vi "Main.vi"(10 "VISA resource name":refnum<visa-resource-name>, 11 "Module Admin":refnum<class "Delacor_lib_QMH_Cloneable Module Admin.lvclass">) -> ()   [LabVIEW 2018, in "Clonable_test.lvlib"]
doc: "This template is based off of the Queued Message Handler design pattern and the Queued Message Handler project template that ships with LabVIEW.\n\nThe main difference is that the queue is private to this module and communication between modules is performed via Broadcast and Request events.\n\nRequest events are wrapped in public API methods and are handled in the Event Handling Loop (EHL) of this VI. Any module can register for Broadcast events sent by this module. The EHL generates messages based on user interface actions.\n\nThe Message Handling Loop (MHL) processes messages generated by the EHL, or by other messages. The messages are string values, so new messages can be added easily to the Message Cases case structure in the MHL. Each message cluster can also provide an optional value for Message Data, which is a variant that can be converted to whatever message-specific data is required.\n_____\nBased on DQMH Project Template 6.0.0.91."
uses:
  Clonable_test.lvlib
  <vilib>/Delacor/Delacor QMH/Libraries/Cloneable Module Admin_class/Delacor_lib_QMH_Cloneable Module Admin.lvclass
  C:/Program Files (x86)/National Instruments/LabVIEW 2018/vi.lib/Delacor/Delacor QMH/Libraries/Module Admin_class/Delacor_lib_QMH_Module Admin.lvclass
  Module Data--cluster.ctl
  <vilib>/Delacor/Delacor QMH/Libraries/Message Queue_class/Delacor_lib_QMH_Message Queue.lvclass/Delacor_lib_QMH_Message Queue.ctl
  <vilib>/Delacor/Delacor QMH/Libraries/Cloneable Module Admin_class/Delacor_lib_QMH_Cloneable Module Admin.lvclass/Delacor_lib_QMH_Cloneable Module Admin.ctl
  Stop Argument--cluster.ctl
  <vilib>/Delacor/Delacor QMH/Libraries/Module Admin_class/Delacor_lib_QMH_Module Admin.lvclass/Delacor_lib_QMH_Module Admin.ctl
  Get data from module Argument--cluster.ctl
  Get data from module (Reply Payload)--cluster.ctl
  start send Argument--cluster.ctl
  stop send Argument--cluster.ctl
  <vilib>/Utility/miscctls.llb/LVPointTypeDef.ctl
  <vilib>/Delacor/Delacor QMH/Libraries/Message Queue_class/Delacor_lib_QMH_Enqueue Message (Single).vi
  <vilib>/Delacor/Delacor QMH/Libraries/Cloneable Module Admin_class/Delacor_lib_QMH_Get Module ID.vi
  <vilib>/Delacor/Delacor QMH/Libraries/Module Admin_class/Delacor_lib_QMH_Get External Launch.vi
  <vilib>/Utility/error.llb/Error Cluster From Error Code.vi
  <vilib>/ErrorRing/Error Ring.xnode
  <vilib>/Delacor/Delacor QMH/Libraries/Message Queue_class/Delacor_lib_QMH_Message Queue.lvclass
panel:
  out "error out":errorcluster
  out "Status":string
  in  "Simulate EHL Error":bool
  in  "Simulate MHL Error":bool
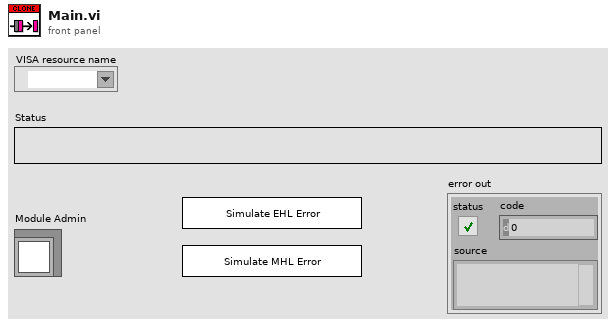
[diagram p1: front panel]
types:
  T1 = typedef "Clonable_test.lvlib/Request Events--cluster.ctl" = cluster{"Stop Module":refnum<user-event>, "Show Panel":refnum<user-event>, "Hide Panel":refnum<user-event>, "Show Diagram":refnum<user-event>, "Get Module Execution Status":refnum<user-event>, "Get data from module":refnum<user-event>, "start send":refnum<user-event>, "stop send":refnum<user-event>}
  T2 = typedef "Clonable_test.lvlib/Module Data--cluster.ctl" = cluster{"Status":string, "VISA resource name":refnum<visa-resource-name>}
  T3 = enum32{"invalid lock state", "Not Locked", "Locked (No Password)", "Password-protected"}
  T4 = typedef "Clonable_test.lvlib/Stop Argument--cluster.ctl" = cluster{"Module ID":i32, "Origin":string, "Exit via Stop Module Req?":bool, "Wait for Module to stop?":bool}
  T5 = typedef "Clonable_test.lvlib/Get data from module Argument--cluster.ctl" = cluster{"Module ID":i32, "Wait Notifier":refnum<notifier>, "wait for reply":bool}
  T6 = typedef "Clonable_test.lvlib/start send Argument--cluster.ctl" = cluster{"Module ID":i32, "Boolean":bool}
  T7 = typedef "Clonable_test.lvlib/stop send Argument--cluster.ctl" = cluster{"Module ID":i32, "Boolean":bool}
  T8 = typedef "LVPointTypeDef.ctl" = cluster{"Horizontal":i16, "Vertical":i16}
  T9 = enum32{"Invalid", "Standard", "Closed", "Hidden", "Minimized", "Maximized"}
  T10 = typedef "Clonable_test.lvlib/Get data from module (Reply Payload)--cluster.ctl" = cluster{"String":string, "Get data from module_error":errorcluster}
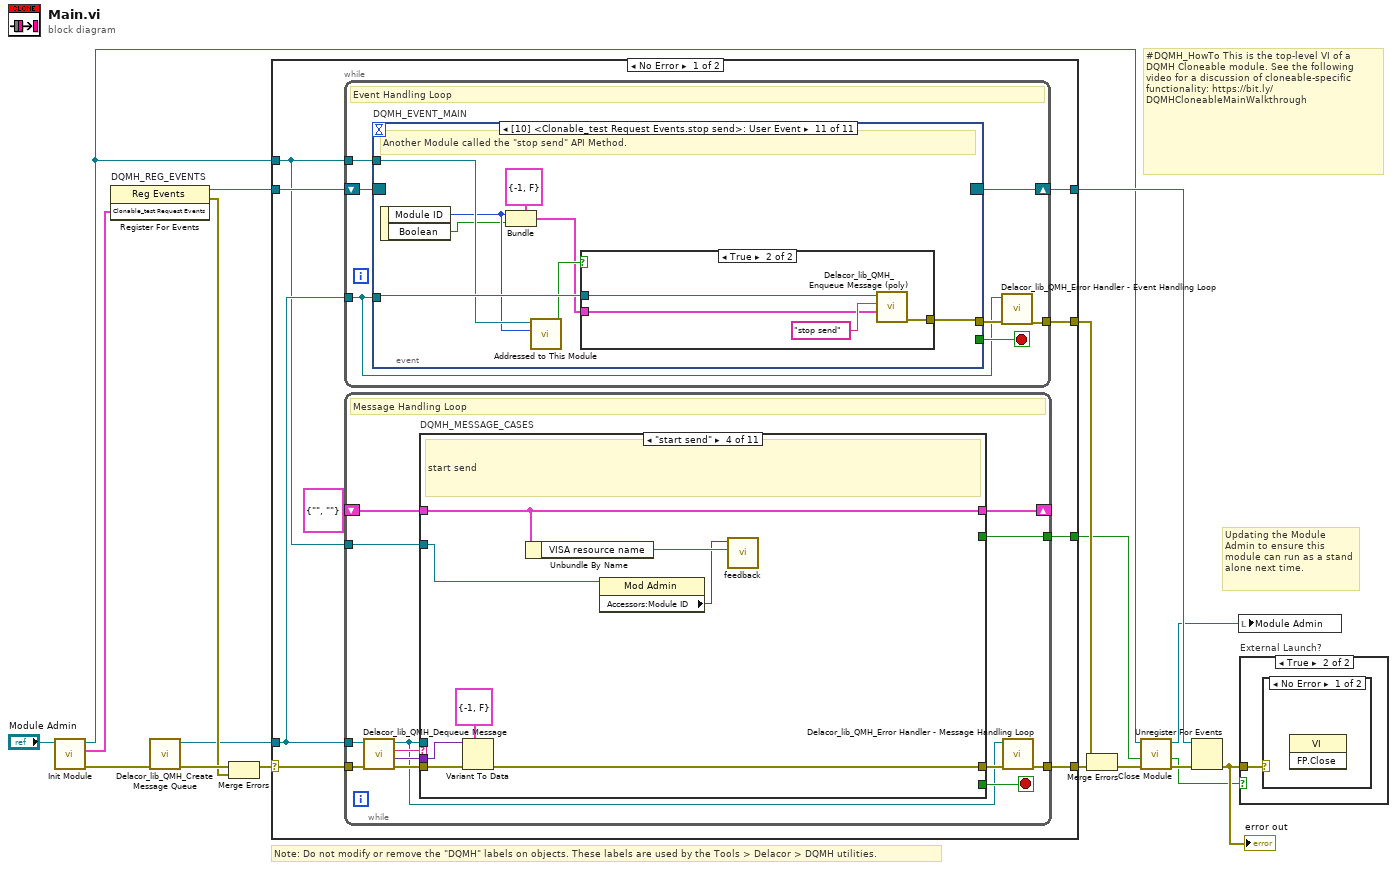
[diagram p0: block diagram]
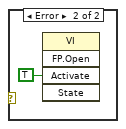
[diagram p3: hidden frame]
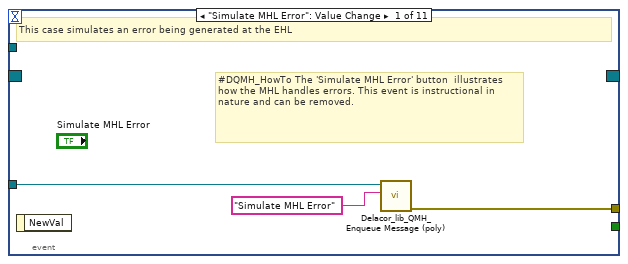
[diagram p4: hidden frame]
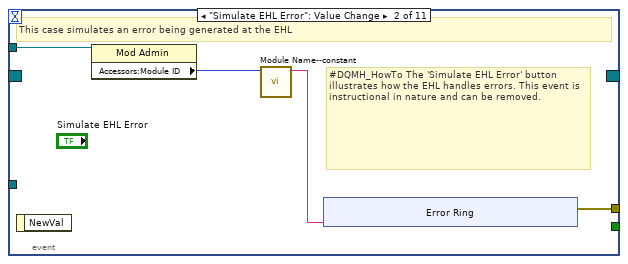
[diagram p5: hidden frame]
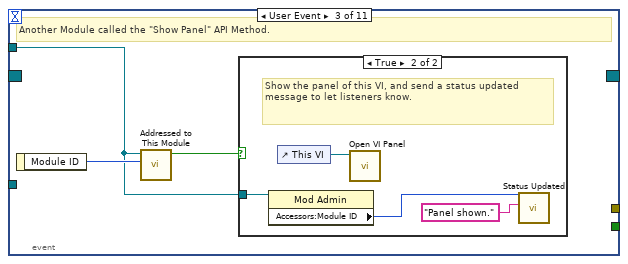
[diagram p6: hidden frame]
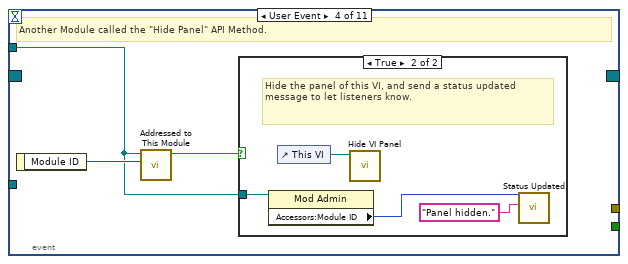
[diagram p8: hidden frame]
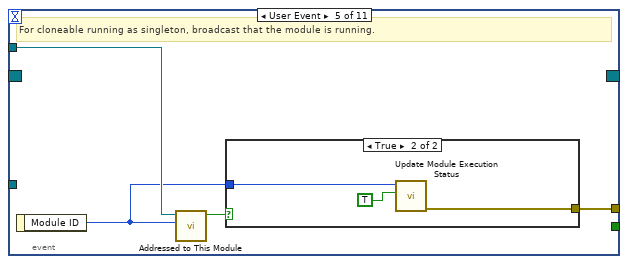
[diagram p10: hidden frame]
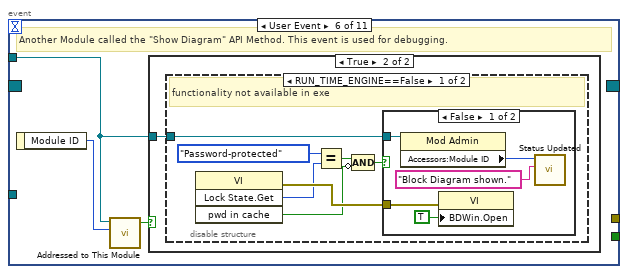
[diagram p12: hidden frame]
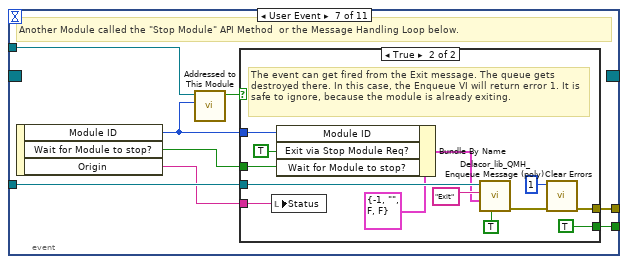
[diagram p16: hidden frame]
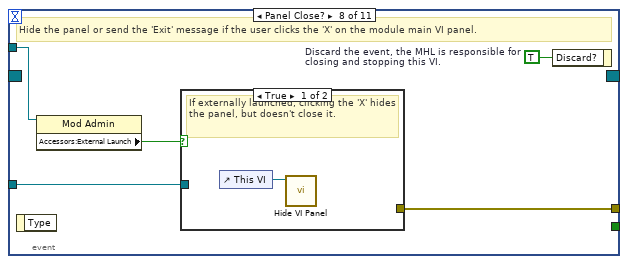
[diagram p18: hidden frame]
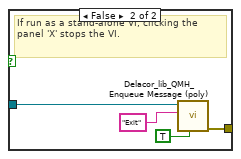
[diagram p19: hidden frame]
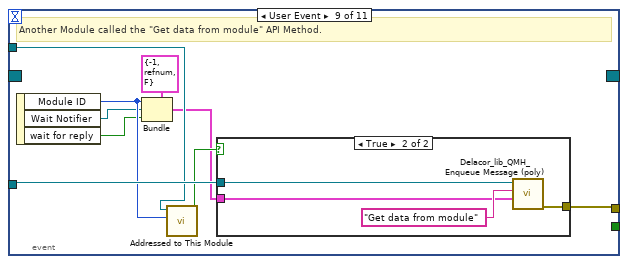
[diagram p20: hidden frame]
diagram:
  # "#DQMH_HowTo This is the top-level VI of a DQMH Cloneable module. See the following video for a discussion of cloneable-specific functionality: https://bit.ly/DQMHCloneableMainWalkthrough"
  # "Note: Do not modify or remove the \"DQMH\" labels on objects. These labels are used by the Tools > Delacor > DQMH utilities."
  # "Updating the Module Admin to ensure this module can run as a stand alone next time."
  n1 = call "Init Module.vi"("Cloneable Module Admin in"="Module Admin") -> ("error out"=w15:errorcluster, "Clonable_test Request Events"=w7:T1, "Cloneable Module Admin out"=w4:refnum<class "Delacor_lib_QMH_Cloneable Module Admin.lvclass">)  [unwired: 8 in]
  n2 = register-events "DQMH_REG_EVENTS"(w7) -> (reference out=w8:refnum<event-registration>, error out=w10:errorcluster)  [unwired: 2 in]
  n3 = call <vilib>:"Delacor_lib_QMH_Create Message Queue.vi"("error in"=w15) -> ("error out"=w12:errorcluster, "Message Queue"=w6:refnum<class "Delacor_lib_QMH_Message Queue.lvclass">)  [unwired: 9 in]
  n4 = Merge Errors(w12, w10) -> (w11:errorcluster)
  n5 = case shown="No Error" w11 {
    selector: w11 -> [w25 w296]
    tunnel: [w27 w295] -> w16
    tunnel: [w24 w303] -> w9
    tunnel: w8 -> [w22 w303]
    tunnel: w6 -> [w21 w294]
    tunnel: [w26 _] -> w17
    tunnel: w4 -> [w20 w299]
    tunnel: [w19 _] -> w2
    frame No Error {
      n6 = while {
        tunnel: w21 -> [w28]
        shift-right: [w31] -> w24
        shift-left: w22 -> [w32]
        tunnel: [w33] -> w26
        tunnel: w20 -> [w29]
        stop <- w30 stop-if-true
        # "Event Handling Loop"
        n7 = event "DQMH_EVENT_MAIN" shown="[10] <Clonable_test Request Events.stop send>: User Event" {
          selector: w32 -> [_ _ _ _ _ _ _ _ _ _ _]
          dyn-events: [_ _ _ _ _ _ _ _ _ _ _] -> w31
          timeout: _ -> [_ _ _ _ _ _ _ _ _ _ _]
          tunnel: [_ _ _ _ _ _ w89 _ _ _ _] -> w30
          tunnel: w28 -> [w36 _ _ _ _ _ w92 w108 w125 w137 w149]
          tunnel: [w37 w41 _ _ w66 _ w93 w111 w117 w130 w142] -> w34
          tunnel: w29 -> [_ w40 w49 w56 w64 w70 w91 w109 w123 w135 w147]
          event "Simulate MHL Error": Value Change {
            # "#DQMH_HowTo The 'Simulate MHL Error' button  illustrates how the MHL handles errors. This event is instructional in nature and can be removed."
            # "This case simulates an error being generated at the EHL"
            n8 = event-data() -> ()  [unwired: 1 in, 1 out]
            n9 = call-poly <vilib>:"Delacor_lib_QMH_Enqueue Message (poly).vi"("Message"="Simulate MHL Error", "Message Queue in"=w36) -> ("error out"=w37:errorcluster)  [unwired: 8 in, 1 out]
          }
          event "Simulate EHL Error": Value Change {
            # "#DQMH_HowTo The 'Simulate EHL Error' button  illustrates how the EHL handles errors. This event is instructional in nature and can be removed."
            # "This case simulates an error being generated at the EHL"
            n10 = event-data() -> ()  [unwired: 1 in, 1 out]
            n11 = property class="Mod Admin"(reference=w40) -> ("Accessors:Module ID"=w39:i32)  [unwired: 1 in, 2 out]
            n12 = call "Module Name--constant.vi"("Module ID"=w39) -> ("Module Name"=w38:string)  [unwired: 10 in]
            n13 = xnode "Error Ring"("parameter 0"=w38) -> ("error out"=w41:errorcluster)
          }
          event User Event {
            # "Another Module called the \"Show Panel\" API Method."
            n14 = event-data() -> ("Module ID"=w50:i32)  [unwired: 1 in]
            n15 = call "Addressed to This Module.vi"("Module ID from Argument"=w50, "Module Admin"=w49) -> ("Addressed to this instance?"=w51:bool)  [unwired: 8 in, 1 out]
            n16 = case shown="True" w51 {
              tunnel: w49 -> [_ w53]
              frame False {
              }
              frame True {
                # "Show the panel of this VI, and send a status updated message to let listeners know."
                n17 = property class="Mod Admin"(reference=w53) -> ("Accessors:Module ID"=w52:i32)  [unwired: 1 in, 2 out]
                n18 = control-ref of="This VI"() -> (w55:refnum<vi>)
                n19 = call "Open VI Panel.vi"("VI"=w55) -> ()  [unwired: 10 in, 1 out]
                n20 = call "Status Updated.vi"("Status"="Panel shown." ("format string"), "Module ID"=w52) -> ()  [unwired: 9 in, 1 out]
              }
            }
          }
          event User Event {
            # "Another Module called the \"Hide Panel\" API Method."
            n21 = event-data() -> ("Module ID"=w57:i32)  [unwired: 1 in]
            n22 = call "Addressed to This Module.vi"("Module ID from Argument"=w57, "Module Admin"=w56) -> ("Addressed to this instance?"=w58:bool)  [unwired: 8 in, 1 out]
            n23 = case shown="True" w58 {
              tunnel: w56 -> [_ w60]
              frame False {
              }
              frame True {
                # "Hide the panel of this VI, and send a status updated message to let listeners know."
                n24 = property class="Mod Admin"(reference=w60) -> ("Accessors:Module ID"=w59:i32)  [unwired: 1 in, 2 out]
                n25 = control-ref of="This VI"() -> (w62:refnum<vi>)
                n26 = call "Hide VI Panel.vi"("VI"=w62) -> ()  [unwired: 10 in, 1 out]
                n27 = call "Status Updated.vi"("Status"="Panel hidden." ("format string"), "Module ID"=w59) -> ()  [unwired: 9 in, 1 out]
              }
            }
          }
          event User Event {
            # "For cloneable running as singleton, broadcast that the module is running."
            n28 = event-data() -> ("Module ID"=w63:i32)  [unwired: 1 in]
            n29 = call "Addressed to This Module.vi"("Module ID from Argument"=w63, "Module Admin"=w64) -> ("Addressed to this instance?"=w65:bool)  [unwired: 8 in, 1 out]
            n30 = case shown="True" w65 {
              tunnel: [_ w69] -> w66
              tunnel: w63 -> [_ w68]
              frame False {
              }
              frame True {
                n31 = call "Update Module Execution Status.vi"("Running?"=TRUE, "Module ID"=w68) -> ("error out"=w69:errorcluster)  [unwired: 9 in]
              }
            }
          }
          event User Event {
            # "Another Module called the \"Show Diagram\" API Method. This event is used for debugging."
            n32 = event-data() -> ("Module ID"=w71:i32)  [unwired: 1 in]
            n33 = call "Addressed to This Module.vi"("Module ID from Argument"=w71, "Module Admin"=w70) -> ("Addressed to this instance?"=w72:bool)  [unwired: 8 in, 1 out]
            n34 = case shown="True" w72 {
              tunnel: w70 -> [_ w73]
              frame False {
              }
              frame True {
                n35 = disable-structure shown="RUN_TIME_ENGINE==False" {
                  disable-tunnel: w73 -> [w74 _]
                  frame condition #0 (active) {
                    # "functionality not available in exe"
                    n36 = invoke class="VI" method="Lock State.Get"() -> (error out=w80:errorcluster, "Get Lock State"=w79:T3, "pwd in cache"=w76:bool)  [unwired: 4 in, 1 out]
                    n37 = Equal?(x=T3."Password-protected", y=w79) -> (x = y?=w77:bool)
                    n38 = Compound Arithmetic op=AND(w77, invert w76) -> (w75:bool)
                    n39 = case shown="False" w75 {
                      tunnel: w80 -> [w85 _]
                      tunnel: w74 -> [w82 _]
                      frame False {
                        n40 = property class="Mod Admin"(reference=w82) -> ("Accessors:Module ID"=w81:i32)  [unwired: 1 in, 2 out]
                        n41 = property class="VI"(error in=w85, "BDWin.Open"=TRUE ("Block Diagram Window:Open")) -> ()  [unwired: 1 in, 2 out]
                        n42 = call "Status Updated.vi"("Status"="Block Diagram shown." ("format string"), "Module ID"=w81) -> ()  [unwired: 9 in, 1 out]
                      }
                      frame True {
                        # "Password-protected VI, and the password is not in the cache. Do not show the diagram."
                      }
                    }
                  }
                  frame condition #1 {
                  }
                }
              }
            }
          }
          event User Event {
            # "Another Module called the \"Stop Module\" API Method  or the Message Handling Loop below."
            n43 = event-data() -> ("Module ID"=w87:i32, "Wait for Module to stop?"=w88:bool, "Origin"=w86:string)  [unwired: 1 in]
            n44 = call "Addressed to This Module.vi"("Module ID from Argument"=w87, "Module Admin"=w91) -> ("Addressed to this instance?"=w90:bool)  [unwired: 8 in, 1 out]
            n45 = case shown="True" w90 {
              tunnel: [_ w105] -> w93
              tunnel: w92 -> [_ w101]
              tunnel: [_ TRUE] -> w89
              tunnel: w88 -> [_ w96]
              tunnel: w87 -> [_ w98]
              tunnel: w86 -> [_ w94]
              frame False {
              }
              frame True {
                # "The event can get fired from the Exit message. The queue gets destroyed there. In this case, the Enqueue VI will return error 1. It is safe to ignore, because the module is already exiting."
                n46 = local write "Status"(w94) -> ()
                n47 = Bundle By Name(cluster=T4 {"Module ID"=-1, "Origin"="", "Exit via Stop Module Req?"=FALSE, "Wait for Module to stop?"=FALSE} ("Stop Argument"), "Module ID"=w98, "Exit via Stop Module Req?"=TRUE, "Wait for Module to stop?"=w96) -> (w95:T4)
                n48 = call-poly <vilib>:"Delacor_lib_QMH_Enqueue Message (poly).vi"("Priority Message? (F)"=TRUE, "Message Data"=w95, "Message"="Exit", "Message Queue in"=w101) -> ("error out"=w106:errorcluster)  [unwired: 6 in, 1 out]
                n49 = call <vilib>:"Clear Errors.vi"("error in (no error)"=w106, "specific error code to clear (0: all)"=1) -> ("error out"=w105:errorcluster)  [unwired: 4 in, 1 out]
              }
            }
          }
          event Panel Close? {
            w110 = TRUE  # Discard the event, the MHL is responsible for closing and stopping this VI.
            # "Hide the panel or send the 'Exit' message if the user clicks the 'X' on the module main VI panel."
            n50 = event-data() -> ()  [unwired: 1 in, 1 out]
            n51 = property class="Mod Admin"(reference=w109) -> ("Accessors:External Launch"=w107:bool)  [unwired: 1 in, 2 out]
            n52 = case shown="True" w107 {
              tunnel: w108 -> [_ w115]
              tunnel: [_ w116] -> w111
              frame True {
                # "If externally launched, clicking the 'X' hides the panel, but doesn't close it."
                n53 = control-ref of="This VI"() -> (w112:refnum<vi>)
                n54 = call "Hide VI Panel.vi"("VI"=w112) -> ()  [unwired: 10 in, 1 out]
              }
              frame False {
                # "If run as a stand-alone VI, clicking the panel 'X' stops the VI."
                n55 = call-poly <vilib>:"Delacor_lib_QMH_Enqueue Message (poly).vi"("Priority Message? (F)"=TRUE, "Message"="Exit", "Message Queue in"=w115) -> ("error out"=w116:errorcluster)  [unwired: 7 in, 1 out]
              }
            }
            n56 = event-data("Discard?"=w110) -> ()  [unwired: 1 in, 1 out]
          }
          event User Event {
            # "Another Module called the \"Get data from module\" API Method."
            n57 = event-data() -> ("Module ID"=w120:i32, "Wait Notifier"=w119:refnum<notifier>, "wait for reply"=w118:bool)  [unwired: 1 in]
            n58 = Bundle(cluster=T5 {"Module ID"=-1, "Wait Notifier"=refnum, "wait for reply"=FALSE} ("Get data from module Argument"), "Module ID"=w120, "Wait Notifier"=w119, "wait for reply"=w118) -> (w121:T5)
            n59 = call "Addressed to This Module.vi"("Module ID from Argument"=w120, "Module Admin"=w123) -> ("Addressed to this instance?"=w124:bool)  [unwired: 8 in, 1 out]
            n60 = case shown="True" w124 {
              tunnel: w125 -> [_ w129]
              tunnel: w121 -> [_ w127]
              tunnel: [_ w126] -> w117
              frame False {
              }
              frame True {
                n61 = call-poly <vilib>:"Delacor_lib_QMH_Enqueue Message (poly).vi"("Message Data"=w127, "Message"="Get data from module", "Message Queue in"=w129) -> ("error out"=w126:errorcluster)  [unwired: 7 in, 1 out]
              }
            }
          }
          event User Event {
            # "Another Module called the \"start send\" API Method."
            n62 = event-data() -> ("Module ID"=w132:i32, "Boolean"=w131:bool)  [unwired: 1 in]
            n63 = Bundle(cluster=T6 {"Module ID"=-1, "Boolean"=FALSE} ("start send Argument"), "Module ID"=w132, "Boolean"=w131) -> (w133:T6)
            n64 = call "Addressed to This Module.vi"("Module ID from Argument"=w132, "Module Admin"=w135) -> ("Addressed to this instance?"=w136:bool)  [unwired: 8 in, 1 out]
            n65 = case shown="True" w136 {
              tunnel: w137 -> [_ w141]
              tunnel: w133 -> [_ w139]
              tunnel: [_ w138] -> w130
              frame False {
              }
              frame True {
                n66 = call-poly <vilib>:"Delacor_lib_QMH_Enqueue Message (poly).vi"("Message Data"=w139, "Message"="start send", "Message Queue in"=w141) -> ("error out"=w138:errorcluster)  [unwired: 7 in, 1 out]
              }
            }
          }
          event User Event {
            # "Another Module called the \"stop send\" API Method."
            n67 = event-data() -> ("Module ID"=w144:i32, "Boolean"=w143:bool)  [unwired: 1 in]
            n68 = Bundle(cluster=T7 {"Module ID"=-1, "Boolean"=FALSE} ("stop send Argument"), "Module ID"=w144, "Boolean"=w143) -> (w145:T7)
            n69 = call "Addressed to This Module.vi"("Module ID from Argument"=w144, "Module Admin"=w147) -> ("Addressed to this instance?"=w148:bool)  [unwired: 8 in, 1 out]
            n70 = case shown="True" w148 {
              tunnel: w149 -> [_ w153]
              tunnel: w145 -> [_ w151]
              tunnel: [_ w150] -> w142
              frame False {
              }
              frame True {
                n71 = call-poly <vilib>:"Delacor_lib_QMH_Enqueue Message (poly).vi"("Message Data"=w151, "Message"="stop send", "Message Queue in"=w153) -> ("error out"=w150:errorcluster)  [unwired: 7 in, 1 out]
              }
            }
          }
        }
        n72 = call-dynamic "Delacor_lib_QMH_Error Handler - Event Handling Loop.vi"("error in"=w34, "Message Queue in"=w28) -> ("dup error in"=w33:errorcluster)  [unwired: 8 in, 1 out]
      }
      n73 = while {
        tunnel: w21 -> [w157]
        shift-right: [w161] -> _
        shift-left: T2 {"Status"="", "VISA resource name"=""} ("Data Cluster") -> [w162]
        tunnel: w25 -> [w165]
        tunnel: [w163] -> w27
        tunnel: w20 -> [w155]
        tunnel: [w154] -> w19
        stop <- w160 stop-if-true
        # "Message Handling Loop"
        n74 = call-dynamic "Delacor_lib_QMH_Dequeue Message.vi"("error in"=w165, "Message Queue in"=w157) -> ("error out"=w164:errorcluster, "Message Data"=w158:variant, "Message"=w159:string, "Message Queue out"=w156:refnum<class "Delacor_lib_QMH_Message Queue.lvclass">)  [unwired: 6 in]
        n75 = case "DQMH_MESSAGE_CASES" shown="\"start send\"" w159 {
          selector: w159 -> [_ _ _ _ _ _ _ _ _ _ w281]
          tunnel: w156 -> [_ _ _ _ _ _ _ w232 _ w271 _]
          tunnel: w164 -> [w187 w191 w209 w219 w225 w228 w230 w241 w254 w277 w283]
          tunnel: [w185 w191 w200 w218 w223 w227 w230 w237 w253 w274 w284] -> w166
          tunnel: w162 -> [w167 w190 w197 w215 w224 w226 w229 w236 w251 w270 w282]
          tunnel: [w178 w190 w197 w215 w224 w226 w229 w236 w251 w270 w282] -> w161
          tunnel: [_ _ _ _ _ _ _ _ _ w269 _] -> w160
          tunnel: w158 -> [_ _ w207 w217 w222 _ _ w235 _ w267 _]
          tunnel: w155 -> [w173 _ _ w213 _ _ _ w234 w249 w263 w279]
          tunnel: [_ _ _ _ _ _ _ _ _ w265 _] -> w154
          frame "Initialize" {
            w170 = "Initial Message" ("Initial Message")
            # "Initialize - Any operation that needs to be done before the module can receive messages. Synchronize Caller Events.vi will inform Start Module.vi that the module has launched and is ready to receive messages. Module Did Init.vi will broadcast that the module initialized."
            n76 = call "Synchronize Caller Events.vi"("error in (no error)"=w187, "Module Admin"=w173) -> ("error out"=w186:errorcluster, "Module Admin out"=w172:refnum<class "Delacor_lib_QMH_Cloneable Module Admin.lvclass">)  [unwired: 8 in]
            n77 = property class="Mod Admin"(reference=w172) -> ("Accessors:Module ID"=w175:i32, "Accessors:External Launch"=w174:bool)  [unwired: 1 in, 2 out]
            n78 = Bundle By Name(cluster=w167, "VISA resource name"="VISA resource name") -> (w168:T2)
            n79 = call "Module Name--constant.vi"("Module ID"=w175) -> ("Module Name"=w182:string)  [unwired: 10 in]
            n80 = property class="VI"("Front Panel.Title"=w182) -> (reference out=w184:refnum<vi>, error out=w189:errorcluster)  [unwired: 2 in]
            n81 = Select(t=T9."Hidden" ("State"), s=w174, f=T9."Standard" ("State")) -> (s? t:f=w179:T9)
            n82 = invoke class="VI" method="FP.Open"(reference=w184, error in=w189, "State"=w179) -> (reference out=w183:refnum<vi>, error out=w188:errorcluster)  [unwired: 2 in, 3 out]
            n83 = call "Module Name--constant.vi"("Module ID"=w175) -> ("Module Name"=w176:string)  [unwired: 10 in]
            n84 = Bundle By Name(cluster=w168, "Status"=w170) -> (w178:T2)
            n85 = invoke class="VI" method="FP.Center"(reference=w183, error in=w188) -> ()  [unwired: 1 in, 3 out]
            n86 = property on="Pane" class="Pane"("Origin"=T8 {"Horizontal"=0, "Vertical"=0}) -> ()  [unwired: 2 in, 2 out]
            n87 = call "Module Did Init.vi"("error in (no error)"=w186, "Initialized?"=TRUE, "Origin"=w176, "Module ID"=w175) -> ("error out"=w185:errorcluster)  [unwired: 7 in]
            "Status" <- w170
          }
          frame "---Module Specific---" {
            # "Separator -- The following cases handle messages specific to this Module."
          }
          frame "Get data from module" {
            # "test function get data from each module"
            n88 = Unbundle By Name(w197) -> ("VISA resource name"=w195:refnum<visa-resource-name>)
            n89 = Variant To Data(error in=w209, type=T5 {"Module ID"=-1, "Wait Notifier"=refnum, "wait for reply"=FALSE} ("Get data from module Argument"), Variant=w207) -> (data=w205:T5, error out=w208:errorcluster)
            n90 = feedback #1(0) -> (w199:i32)
            n91 = Increment(x=w199) -> (x+1=w194:i32)
            n92 = feedback-in #1(w194) -> ()
            n93 = Unbundle By Name(w205) -> ("Wait Notifier"=w204:refnum<notifier>, "wait for reply"=w203:bool)  [unwired: 1 out]
            n94 = Format Into String(format string="%d: %s\\n", w194, w195) -> (resulting string=w193:string, error out=w192:errorcluster)  [unwired: 2 in]
            n95 = Bundle By Name(cluster=T10 {"String"="", "Get data from module_error"={"status"=FALSE, "code"=0, "source"=""}} ("Get data from module (Reply Payload)"), "String"=w193, "Get data from module_error"=w192) -> (w202:T10)
            n96 = case shown="True" w203 {
              tunnel: w204 -> [_ w211]
              tunnel: w202 -> [_ w210]
              frame False {
              }
              frame True {
                n97 = Send Notification(notification=w210, notifier=w211) -> ()  [unwired: 1 in, 2 out]
              }
            }
            n98 = Merge Errors(w208, w192) -> (w200:errorcluster)
          }
          frame "start send" {
            # "start send"
            n99 = Variant To Data(error in=w219, type=T6 {"Module ID"=-1, "Boolean"=FALSE} ("start send Argument"), Variant=w217) -> (error out=w218:errorcluster)  [unwired: 1 out]
            n100 = Unbundle By Name(w215) -> ("VISA resource name"=w214:refnum<visa-resource-name>)
            n101 = property class="Mod Admin"(reference=w213) -> ("Accessors:Module ID"=w212:i32)  [unwired: 1 in, 2 out]
            n102 = call "feedback.vi"("String"=w214, "Module ID"=w212) -> ()  [unwired: 9 in, 1 out]
          }
          frame "stop send" {
            # "#CodeNeeded\n1. Configure this Message Case for handling the \"stop send\" message.\n2. Delete or edit this label when done."
            n103 = Variant To Data(error in=w225, type=T7 {"Module ID"=-1, "Boolean"=FALSE} ("stop send Argument"), Variant=w222) -> (data=w220:T7, error out=w223:errorcluster)
            n104 = Unbundle By Name(w220) -> ()  [unwired: 2 out]
          }
          frame "---Copy This Frame---" {
            # "Duplicate this frame when creating new messages.  Change this comment in the duplicated frame to describe this message."
            n105 = Merge Errors(w228) -> (w227:errorcluster)
          }
          frame "---Exit and Error Handling---" {
            # "Separator - the following cases handle errors and exit messages."
          }
          frame "Error" {
            # "#CodeRecommended - If you ever change the name of this \"Error\" message, you'll need to update the name in the Check Loop Error.vi as well."
            # "#CodeRecommended - If the module is running in standalone mode (External Launch = FALSE), this code will pop up an error dialog and call the 'Exit' message if an error occurs. Add more fine-grained error handling here."
            # "Error - Check the error message data and respond accordingly. This message is sent by the \"Error Handler\" VIs at the end of each loop in this application."
            n106 = property class="Mod Admin"(reference=w234) -> ("Accessors:External Launch"=w233:bool, "Accessors:Module ID"=w231:i32)  [unwired: 1 in, 2 out]
            n107 = Variant To Data(error in=w241, type=errorcluster {"status"=FALSE, "code"=0, "source"=""} ("error constant"), Variant=w235) -> (data=w242:errorcluster, error out=w239:errorcluster)
            n108 = call "Error Reported.vi"("Error"=w242, "Module ID"=w231) -> ()  [unwired: 9 in, 1 out]
            n109 = case shown="False" w233 {
              tunnel: [w247 _] -> w238
              tunnel: w232 -> [w245 _]
              tunnel: w242 -> [w246 _]
              frame False {
                # "If the module is running standalone, then pop up an error dialog and call the \"Exit\" message."
                n110 = call <vilib>:"Simple Error Handler.vi"("error in (no error)"=w246) -> ()  [unwired: 4 in, 5 out]
                n111 = call-poly <vilib>:"Delacor_lib_QMH_Enqueue Message (poly).vi"("Priority Message? (F)"=TRUE, "Message"="Exit", "Message Queue in"=w245) -> ("error out"=w247:errorcluster)  [unwired: 7 in, 1 out]
              }
              frame True {
                # "If the module was launched externally, calling the Error Reported broadcast VI is the only action performed by the \"Error\" message. The module's caller can then process the error appropriately."
              }
            }
            n112 = Merge Errors(w239, w238) -> (w237:errorcluster)
            n113 = local write "error out"(w237) -> ()
          }
          frame "Simulate MHL Error" {
            # "#DQMH_HowTo The 'Simulate MHL Error' button  illustrates how the MHL handles errors. This event is instructional in nature and can be removed."
            # "Simulate an error occurring at the MHL"
            n114 = property class="Mod Admin"(reference=w249) -> ("Accessors:Module ID"=w250:i32)  [unwired: 1 in, 2 out]
            n115 = call "Module Name--constant.vi"("Module ID"=w250) -> ("Module Name"=w248:string)  [unwired: 10 in]
            n116 = xnode "Error Ring"("parameter 0"=w248) -> ("error out"=w252:errorcluster)
            n117 = Merge Errors(w254, w252) -> (w253:errorcluster)
          }
          frame "Exit" {
            w268 = 91  # 91: not all Exit messages will have an argument
            w269 = TRUE  # Stop the VI
            # "Release the message queue reference"
            # "#CodeNeeded - Add any required cleanup code here."
            # "Exit - Exit the application."
            n118 = Variant To Data(error in=w277, type=T4 {"Module ID"=-1, "Origin"="", "Exit via Stop Module Req?"=FALSE, "Wait for Module to stop?"=FALSE} ("Stop Argument"), Variant=w267) -> (data=w264:T4, error out=w272:errorcluster)
            n119 = call <vilib>:"Clear Errors.vi"("error in (no error)"=w272, "specific error code to clear (0: all)"=w268) -> ("error out"=w276:errorcluster)  [unwired: 4 in, 1 out]
            n120 = control-ref of="This VI"() -> (w262:refnum<vi>)
            n121 = call-dynamic "Delacor_lib_QMH_Release Message Queue.vi"("error in"=w276, "Message Queue"=w271) -> ("error out"=w275:errorcluster)  [unwired: 9 in]
            n122 = call "Handle Exit.vi"("Stop Argument"=w264, "Module Admin in"=w263, "VI reference"=w262) -> ("error out"=w273:errorcluster, "Wait for Stop?"=w265:bool)  [unwired: 7 in]
            n123 = Merge Errors(w275, w273) -> (w274:errorcluster)
          }
          frame Default {
            # "'Default' case only runs if there is a message that isn't defined in any of the other cases.  Output a programming error."
            n124 = property class="Mod Admin"(reference=w279) -> ("Accessors:Module ID"=w278:i32)  [unwired: 1 in, 2 out]
            n125 = call "Module Name--constant.vi"("Module ID"=w278) -> ("Module Name"=w280:string)  [unwired: 10 in]
            n126 = xnode "Error Ring"("parameter 0"=w281, "parameter 1"=w280) -> ("error out"=w285:errorcluster)
            n127 = Merge Errors(w283, w285) -> (w284:errorcluster)
          }
        }
        n128 = call-dynamic "Delacor_lib_QMH_Error Handler - Message Handling Loop.vi"("error in"=w166, "Message Queue in"=w156) -> ("dup error in"=w163:errorcluster)  [unwired: 8 in, 1 out]
      }
    }
    frame Error {
      n129 = call "Synchronize Caller Events.vi"("Module Admin"=w299) -> ("Module Admin out"=w298:refnum<class "Delacor_lib_QMH_Cloneable Module Admin.lvclass">)  [unwired: 9 in, 1 out]
      n130 = property class="Mod Admin"(reference=w298) -> ("Accessors:Module ID"=w297:i32)  [unwired: 1 in, 2 out]
      n131 = call-dynamic "Delacor_lib_QMH_Release Message Queue.vi"("error in"=w296, "Message Queue"=w294) -> ("error out"=w295:errorcluster)  [unwired: 9 in]
      n132 = call "Module Name--constant.vi"("Module ID"=w297) -> ("Module Name"=w302:string)  [unwired: 10 in]
      n133 = Format Into String(format string="An error occurred during initialization. %s is no longer running.", w302) -> (resulting string=w300:string)  [unwired: 2 in, 1 out]
      n134 = call "Error Reported.vi"("Additional Information"=w300, "Error"=w295, "Module ID"=w297) -> ()  [unwired: 8 in, 1 out]
    }
  }
  n135 = Merge Errors(w17, w16) -> (w18:errorcluster)
  n136 = call "Close Module.vi"("error in"=w18, "Wait for stop?"=w2, "Module Admin in"=w4) -> ("error out"=w14:errorcluster, "External Launch"=w1:bool, "Module Admin out"=w3:refnum<class "Delacor_lib_QMH_Cloneable Module Admin.lvclass">)  [unwired: 6 in]
  n137 = Unregister For Events(event registration refnum=w9, error in=w14) -> (error out=w13:errorcluster)
  "error out" <- w13
  n138 = local write "Module Admin"(w3) -> ()
  n139 = case "External Launch?" shown="True" w1 {
    tunnel: w13 -> [_ w304]
    frame False {
    }
    frame True {
      n140 = case shown="No Error" w304 {
        frame No Error {
          n141 = invoke class="VI" method="FP.Close"() -> ()  [unwired: 3 in, 3 out]
        }
        frame Error {
          n142 = invoke class="VI" method="FP.Open"("Activate"=TRUE ("Activate?")) -> ()  [unwired: 4 in, 5 out]
        }
      }
    }
  }
